vi "Set preferenze grafici.vi"() -> (2 "ANNULLA":bool, 3 "GRAPH":refnum<vi>)   [LabVIEW 2019]
panel:
  in  "ANNULLA":bool
  in  "OK":bool
  out "CURVE IDRAULICHE QH":cluster{"X":dbl[], "Y":dbl[]}[](graph)
  # "IMPOSTA PREFERENZE PER TUTTI I GRAFICI"
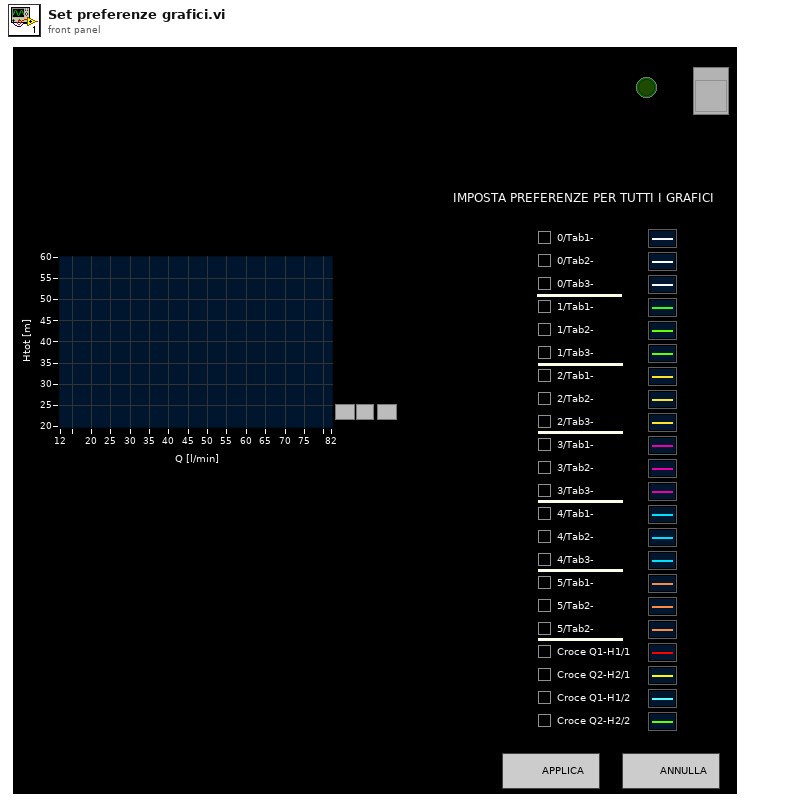
[diagram p1: front panel]
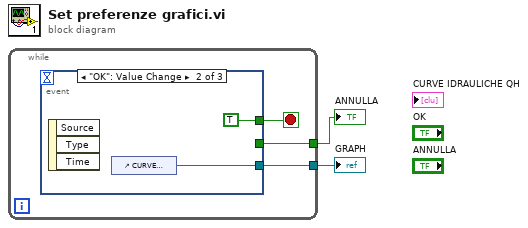
[diagram p0: block diagram]
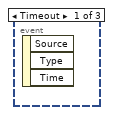
[diagram p2: hidden frame]
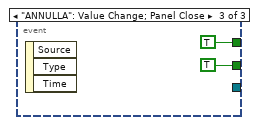
[diagram p3: hidden frame]
diagram:
  n1 = while {
    tunnel: [w4] -> w2
    tunnel: [w3] -> w1
    stop <- w5 stop-if-true
    n2 = event shown="[1] \"OK\": Value Change" {
      selector: _ -> [_ _ _]
      dyn-events: _ -> [_ _ _]
      timeout: _ -> [_ _ _]
      tunnel: [_ TRUE TRUE] -> w5
      tunnel: [_ _ TRUE] -> w4
      tunnel: [_ w6 _] -> w3
      event Timeout {
        n3 = event-data() -> ()  [unwired: 1 in, 3 out]
      }
      event "OK": Value Change {
        n4 = event-data() -> ()  [unwired: 1 in, 3 out]
        n5 = control-ref of="CURVE IDRAULICHE QH"() -> (w6:refnum<vi>)
      }
      event "ANNULLA": Value Change; Panel Close {
        n6 = event-data() -> ()  [unwired: 1 in, 3 out]
      }
    }
  }
  "ANNULLA" <- w2
  "GRAPH" <- w1
